vi "New.vi"(8 "error in (no error)":errorcluster, 11 "File Path":path) -> (0 "error out":errorcluster, 3 "File Sink out":refnum<class "File Sink.lvclass">)   [LabVIEW 2020, in "LV Logging.lvlib" / "File Sink.lvclass"]
uses:
  File Sink.lvclass
  File Sink.lvclass/File Sink.ctl
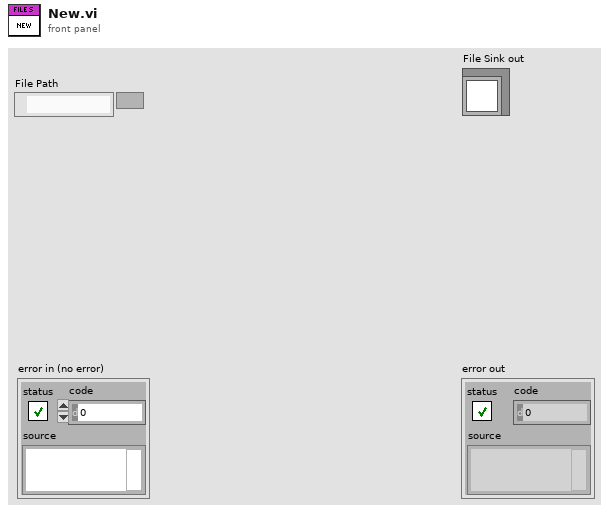
[diagram p1: front panel]
types:
  T1 = enum16{"open", "replace", "create", "open or create", "replace or create", "replace or create with confirmation"}
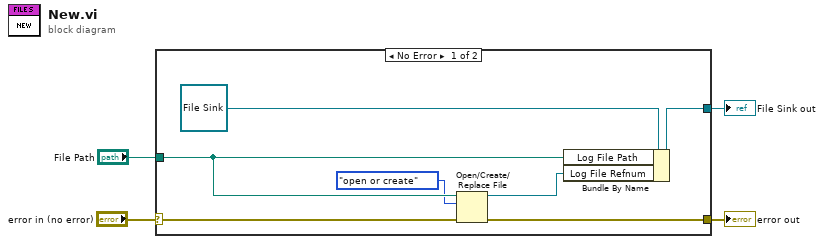
[diagram p0: block diagram]
diagram:
  n1 = case shown="No Error" "error in (no error)" {
    selector: "error in (no error)" -> [w6 w12]
    tunnel: [w9 w12] -> w3
    tunnel: [w10 _] -> w2
    tunnel: "File Path" -> [w8 _]
    frame No Error {
      n2 = Open/Create/Replace File(file path (use dialog)=w8, error in=w6, operation (0:open)=T1."open or create") -> (refnum out=w5:refnum<file>, error out=w9:errorcluster)  [unwired: 3 in, 1 out]
      n3 = Bundle By Name(cluster=refnum<class "File Sink.lvclass"> refnum ("File Sink in"), "Log File Path"=w8, "Log File Refnum"=w5) -> (w10:refnum<class "File Sink.lvclass">)
    }
    frame Error {
    }
  }
  "error out" <- w3
  "File Sink out" <- w2
